vi "DurationToMB.vi"(1 "Experiment Duration (hr)":u16=20, 2 "fs (hz)":u16) -> (0 "FileSize(MB)":i16)   [LabVIEW 2017]
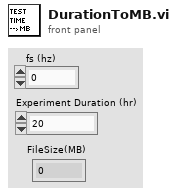
[diagram p1: front panel]
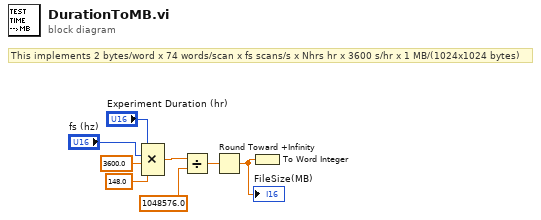
[diagram p0: block diagram]
diagram:
  # "This implements 2 bytes/word x 74 words/scan x fs scans/s x Nhrs hr x 3600 s/hr x 1 MB/(1024x1024 bytes)"
  n1 = Compound Arithmetic op=MULTIPLY("Experiment Duration (hr)", "fs (hz)", 3600.0 ("value"), 148.0 ("value")) -> (w5:dbl)
  n2 = Divide(x=w5, y=1048576.0) -> (x/y=w3:dbl)
  n3 = Round Toward +Infinity(x=w3) -> (ceil(x): smallest int >= x=w2:dbl)
  "FileSize(MB)" <- w2
  n4 = To Word Integer(number=w2) -> ()  [unwired: 1 out]
